vi "CalculateToRef.vi"(10 "New Data":dbl[][](array[numeric]), 11 "Old Data":dbl[][](array[numeric])) -> (2 "Amlitude":dbl[](array[numeric]), 3 "Frequency":dbl[](array[numeric]))   [LabVIEW 2021]
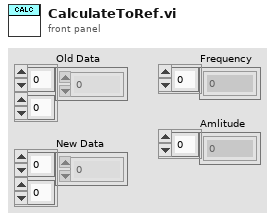
[diagram p1: front panel]
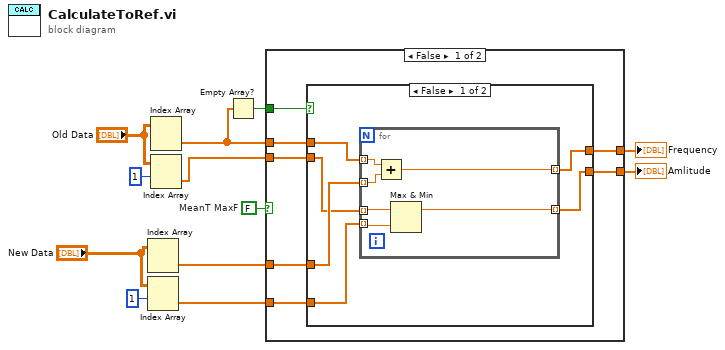
[diagram p0: block diagram]
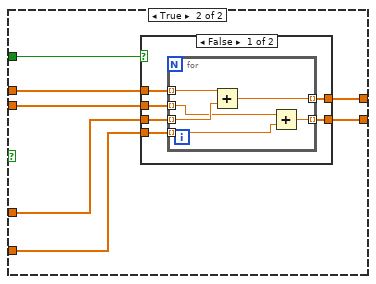
[diagram p3: hidden frame]
diagram:
  w2 = FALSE  # MeanT MaxF
  n1 = Index Array(array="New Data") -> (element=w4:dbl[])  [unwired: 2 in]
  n2 = Index Array(array="New Data", index (row)=1) -> (element=w10:dbl[])  [unwired: 1 in]
  n3 = Index Array(array="Old Data") -> (element=w3:dbl[])  [unwired: 2 in]
  n4 = Index Array(array="Old Data", index (row)=1) -> (element=w5:dbl[])  [unwired: 1 in]
  n5 = Empty Array?(array=w3) -> (empty?=w1:bool)
  n6 = case shown="False" w2 {
    tunnel: [w15 w40] -> w12
    tunnel: [w16 w39] -> w11
    tunnel: w10 -> [w17 w38]
    tunnel: w5 -> [w13 w37]
    tunnel: w4 -> [w18 w36]
    tunnel: w3 -> [w14 w35]
    tunnel: w1 -> [w19 w34]
    frame False {
      n7 = case shown="False" w19 {
        tunnel: w18 -> [w24 w33]
        tunnel: w17 -> [w21 w32]
        tunnel: [w23 w33] -> w16
        tunnel: [w20 w32] -> w15
        tunnel: w14 -> [w25 _]
        tunnel: w13 -> [w22 _]
        frame False {
          n8 = for {
            tunnel: w25 -> [w31] mode=indexing
            tunnel: w24 -> [w30] mode=indexing
            tunnel: [w29] -> w23 mode=indexing
            tunnel: w22 -> [w28] mode=indexing
            tunnel: w21 -> [w27] mode=indexing
            tunnel: [w26] -> w20 mode=indexing
            n9 = Add(x=w31, y=w30) -> (x+y=w29:dbl)
            n10 = Max & Min(x=w28, y=w27) -> (max(x,y)=w26:dbl)  [unwired: 1 out]
          }
        }
        frame True {
        }
      }
    }
    frame True {
      n11 = case shown="False" w34 {
        tunnel: [w46 w53] -> w40
        tunnel: [w45 w54] -> w39
        tunnel: w38 -> [w44 w53]
        tunnel: w37 -> [w43 _]
        tunnel: w36 -> [w42 w54]
        tunnel: w35 -> [w41 _]
        frame False {
          n12 = for {
            tunnel: w41 -> [w52] mode=indexing
            tunnel: w43 -> [w50] mode=indexing
            tunnel: w42 -> [w51] mode=indexing
            tunnel: w44 -> [w49] mode=indexing
            tunnel: [w48] -> w45 mode=indexing
            tunnel: [w47] -> w46 mode=indexing
            n13 = Add(x=w52, y=w51) -> (x+y=w48:dbl)
            n14 = Add(x=w50, y=w49) -> (x+y=w47:dbl)
          }
        }
        frame True {
        }
      }
    }
  }
  "Amlitude" <- w12
  "Frequency" <- w11
